vi "DriveDual.vi"(9 "YAxis":dbl, 10 "XAxis":dbl) -> (2 "Right":dbl, 3 "Left":dbl)   [LabVIEW 2017]
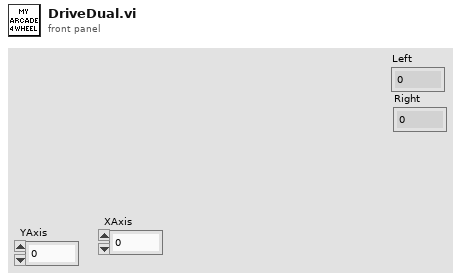
[diagram p1: front panel]
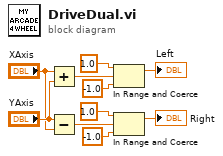
[diagram p0: block diagram]
diagram:
  n1 = Add(x="XAxis", y="YAxis") -> (x+y=w8:dbl)
  n2 = Subtract(x="YAxis", y="XAxis") -> (x-y=w3:dbl)
  n3 = In Range and Coerce(upper limit=1.0, x=w8, lower limit=-1.0) -> (coerced(x)=→"Left":dbl)  [unwired: 1 out]
  n4 = In Range and Coerce(upper limit=1.0, x=w3, lower limit=-1.0) -> (coerced(x)=→"Right":dbl)  [unwired: 1 out]
